vi "Reset stages speed.vi"(8 "error in (no error)":errorcluster, 11 "Autofocus in":refnum<class "Autofocus.lvclass">) -> (0 "error out":errorcluster, 3 "Autofocus out":refnum<class "Autofocus.lvclass">)   [LabVIEW 2012, in "Autofocus.lvclass"]
uses:
  Autofocus.lvclass
  <vilib>/Distrio/Murmex/Murmex/update_cluster.ctl
  Autofocus.lvclass/Autofocus.ctl
  <vilib>/Distrio/Murmex/Murmex/Murmex.lvclass
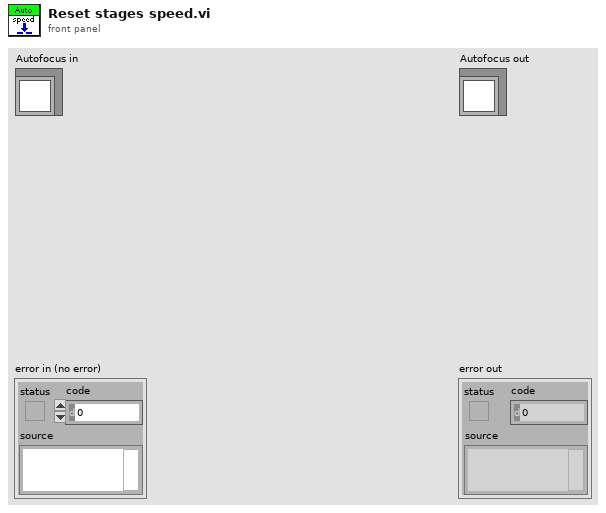
[diagram p1: front panel]
types:
  T1 = typedef "Murmex.lvlib/Murmex.lvclass/update_cluster.ctl" = cluster{"target ID":string, "key chains":string[], "values":variant[]}
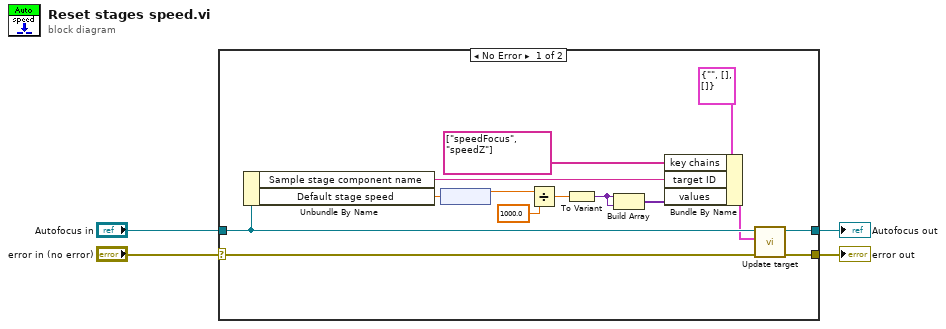
[diagram p0: block diagram]
diagram:
  n1 = case shown="No Error" "error in (no error)" {
    selector: "error in (no error)" -> [w18 w20]
    tunnel: [w17 w20] -> w3
    tunnel: [w16 w19] -> w1
    tunnel: "Autofocus in" -> [w15 w19]
    frame No Error {
      n2 = Unbundle By Name(w15) -> ("Sample stage component name"=w12:string, "Default stage speed"=w10:dbl[unit])
      n3 = node(w10) -> (w9:dbl)
      n4 = Divide(x=w9, y=1000.0) -> (x/y=w7:dbl)
      n5 = To Variant(anything=w7) -> (Variant=w5:variant)
      n6 = Build Array(w5, w5) -> (w6:variant[])
      n7 = Bundle By Name(cluster=T1 {"target ID"="", "key chains"=[], "values"=[]} ("update cluster"), "key chains"=string[] ["speedFocus", "speedZ"], "target ID"=w12, "values"=w6) -> (w13:T1)
      n8 = call <vilib>:"Update target.vi"("error in (no error)"=w18, "update cluster"=w13, "MurmexBase in"=w15) -> ("error out"=w17:errorcluster, "MurmexBase out"=w16:refnum<class "Autofocus.lvclass">)  [unwired: 7 in]
    }
    frame Error {
    }
  }
  "error out" <- w3
  "Autofocus out" <- w1
